vi "Add rate.vi"(8 "error in (no error)":errorcluster, 11 "Automatic Mode in":refnum<class "Automatic Mode.lvclass">) -> (0 "error out":errorcluster, 3 "Automatic Mode out":refnum<class "Automatic Mode.lvclass">)   [LabVIEW 2015, in "Automatic Mode.lvclass"]
uses:
  Automatic Mode.lvclass
  Automatic Mode.lvclass/Automatic Mode.ctl
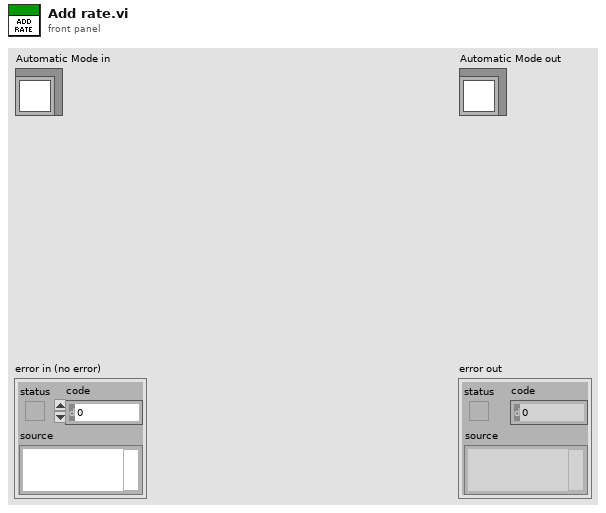
[diagram p1: front panel]
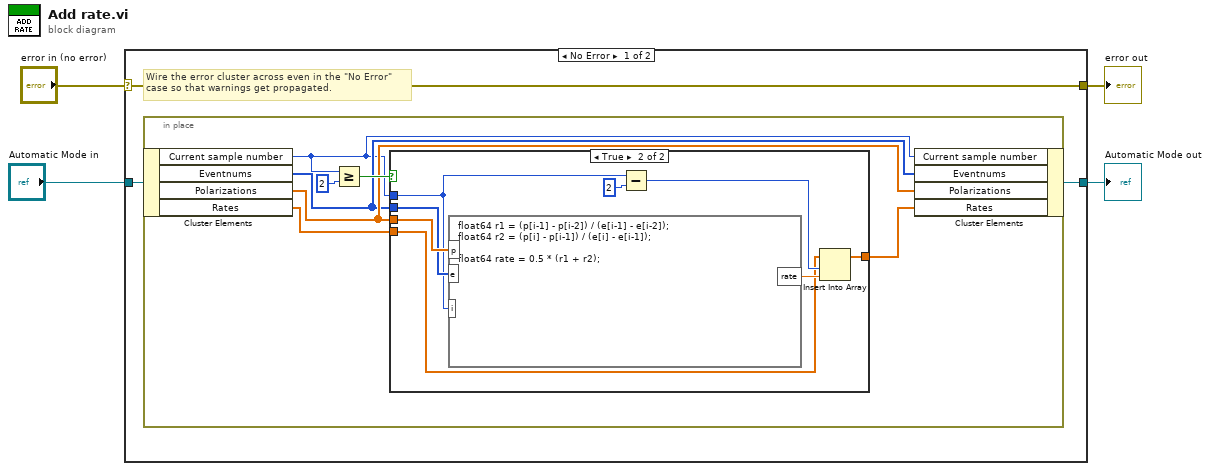
[diagram p0: block diagram]
diagram:
  n1 = case shown="No Error" "error in (no error)" {
    selector: "error in (no error)" -> [w7 w25]
    tunnel: [w7 w25] -> w3
    tunnel: [w5 w24] -> w1
    tunnel: "Automatic Mode in" -> [w6 w24]
    frame No Error {
      # "Wire the error cluster across even in the \"No Error\"\ncase so that warnings get propagated."
      n2 = in-place {
        n3 = in-place-cluster #1(w6) -> ("Current sample number"=w8:i32, "Eventnums"=w9:i64[], "Polarizations"=w10:dbl[], "Rates"=w12:dbl[])
        n4 = Greater Or Equal?(x=w8, y=2) -> (x >= y?=w13:bool)
        n5 = case shown="True" w13 {
          tunnel: w10 -> [_ w23]
          tunnel: w9 -> [_ w22]
          tunnel: w8 -> [_ w20]
          tunnel: w12 -> [w15 w17]
          tunnel: [w15 w16] -> w11
          frame False {
          }
          frame True {
            n6 = formula code="float64 r1 = (p[i-1] - p[i-2]) / (e[i-1] - e[i-2]);\nfloat64 r2 = (p[i] - p[i-1]) / (e[i] - e[i-1]);\n\nfloat64 rate = 0.5 * (r1 + r2);"("p"=w23, "e"=w22, "i"=w20) -> ("rate"=w21:dbl)
            n7 = Subtract(x=w20, y=2) -> (x-y=w18:i32)
            n8 = Insert Into Array(array=w17, index=w18, new element=w21) -> (w16:dbl[])
          }
        }
        n9 = in-place-cluster #1("Current sample number"=w8, "Eventnums"=w9, "Polarizations"=w10, "Rates"=w11) -> (w5:refnum<class "Automatic Mode.lvclass">)
      }
    }
    frame Error {
    }
  }
  "error out" <- w3
  "Automatic Mode out" <- w1
